vi "write sdf ref.vi"(8 "error in (no error)":errorcluster, 10 "sdf ref":refnum<k24>, 11 "abstract-tree in":refnum<class "abstract-tree.lvclass">) -> (0 "error out":errorcluster, 3 "abstract-tree out":refnum<class "abstract-tree.lvclass">)   [LabVIEW 2017, in "vs-tree-utility.lvlib" / "abstract-tree.lvclass"]
uses:
  abstract-tree.lvclass
  NationalInstruments.VeriStand.SystemDefinitionAPI
  abstract-tree.lvclass/abstract-tree.ctl
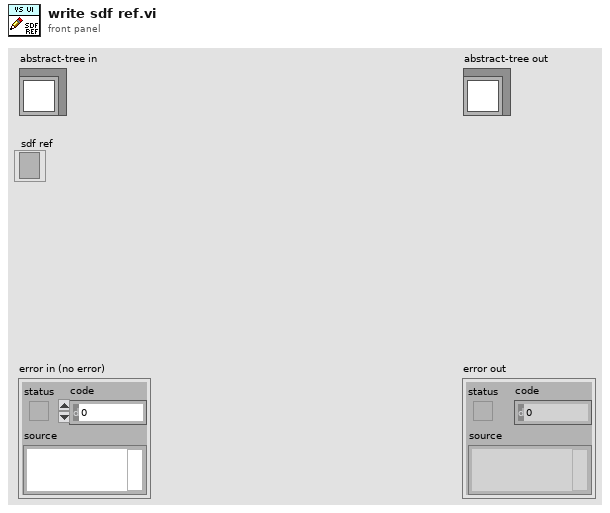
[diagram p1: front panel]
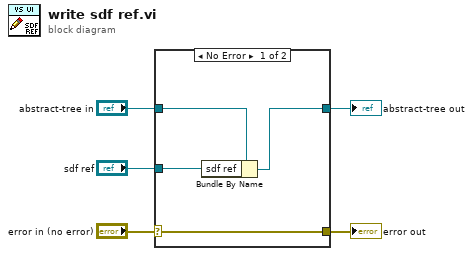
[diagram p0: block diagram]
diagram:
  n1 = case shown="No Error" "error in (no error)" {
    selector: "error in (no error)" -> [w9 w11]
    tunnel: [w9 w11] -> w4
    tunnel: [w7 w10] -> w2
    tunnel: "abstract-tree in" -> [w8 w10]
    tunnel: "sdf ref" -> [w6 _]
    frame No Error {
      n2 = Bundle By Name(cluster=w8, "sdf ref"=w6) -> (w7:refnum<class "abstract-tree.lvclass">)
    }
    frame Error {
    }
  }
  "error out" <- w4
  "abstract-tree out" <- w2
